vi "SmartUsageOfPropertyNode.vi"() -> ()   [LabVIEW 2019]
panel:
  in  "stop":bool
  in  "Numeric":dbl
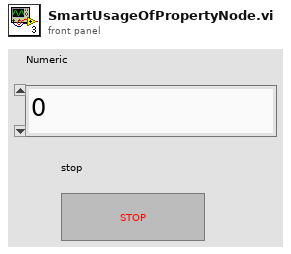
[diagram p1: front panel]
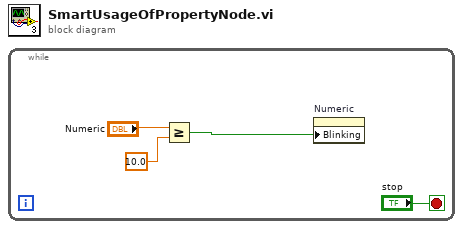
[diagram p0: block diagram]
diagram:
  n1 = while {
    stop <- "stop" stop-if-true
    n2 = Greater Or Equal?(x="Numeric", y=10.0) -> (x >= y?=w2:bool)
    n3 = property on="Numeric" class="DigNum (strict)"("Blinking"=w2) -> ()  [unwired: 2 in, 2 out]
  }
